vi "CompareReadResults.vi"() -> ()   [LabVIEW 2018]
panel:
  out "Waveform Graph":dbl[][](graph)
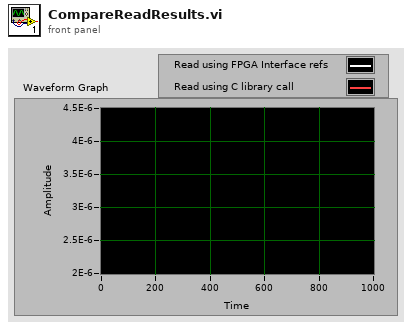
[diagram p1: front panel]
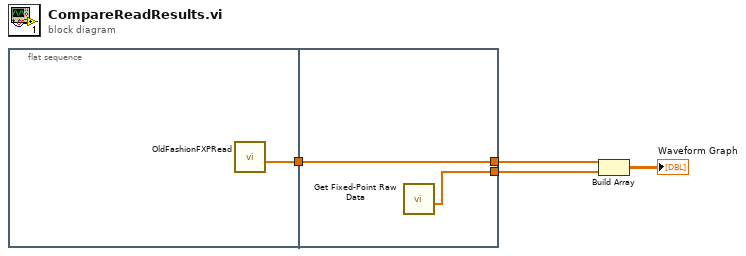
[diagram p0: block diagram]
diagram:
  n1 = flat-sequence {
    tunnel: [w5] -> w3
    tunnel: [w7] -> w4
    tunnel: w3 -> [w7]
    tunnel: [w6] -> w2
    frame #0 {
      n2 = call "OldFashionFXPRead.vi"() -> ("Values"=w5:dbl[])  [unwired: 9 in, 2 out]
    }
    frame #1 {
      n3 = call "Get Fixed-Point Raw Data.vi"() -> ("Values"=w6:dbl[])  [unwired: 10 in, 1 out]
    }
  }
  n4 = Build Array(w4, w2) -> (→"Waveform Graph":dbl[][])
